vi "viewer.vi"() -> ()   [LabVIEW 2018]
uses:
  Status.ctl
  <vilib>/vision/Avi.llb/IMAQ AVI2 Refnum.ctl
  <vilib>/vision/Image Controls.llb/IMAQ Image.ctl
  Temp/gpm_realsense_videos/Converted/ROI STYP.ctl
  <userlib>/Jet Engineering/JET_QSM/Code/Private/JET_QSM_InvalidOption STYP.ctl
  <vilib>/vision/Avi.llb/IMAQ AVI2 Codec Path.ctl
  <userlib>/Jet Engineering/JET_QSM/Code/Private/JET_QSM - Add State [String API].vi
  <userlib>/Jet Engineering/JET_QSM/Code/Private/JET_QSM - Add State to Front [String API].vi
  <vilib>/Utility/error.llb/Trim Whitespace.vi
  <vilib>/Utility/error.llb/Error Cluster From Error Code.vi
  <vilib>/vision/NI_Vision_Development_Module.lvlib
panel:
  in  "Filter Parameters":T1={"Sigma"=1.0, "HThresh"=0.7, "LThres"=0.2, "WindowSize"=9} {"LThres" min=0 max=1 format="%.2f"; "HThresh" min=0 max=1 format="%.2f"; "Sigma" min=0 max=1 format="%.2f"}
  out "Waveform Graph":u32[][](graph)
  in  "Adjust Filtering Options":bool
  in  "Loop?":bool
  in  "Apply Filtering?":bool
  in  "select roi":bool
  in  "ROI Type":T2
  in  "Exit":bool
  out "playback position":dbl(slide) scale=0.0..100.0
  in  "stop":bool
  in  "Start?":bool
  out "Image":T3(plugin-control)
  in  "Video Path":path
  out "Recent states before Error (with tick counts) 2":string="0.167 sec ago: VI Initialize\n0.167 sec ago: Window Open\n0.110 sec ago: Control Update\n0.110 sec ago: Indicator Update\n0.000 sec ago: Error Handler\r\n"
  in  "Status":T4={"VI"={"error"={"status"=FALSE, "code"=0, "source"=""}, "isExiting?"=FALSE}, "UserLoggedIn?"=FALSE, "AVI Refnum"=refnum, "video path"=path "", "Frame Data"={"Width"=0, "Height"=0, "Frames Per Second"=0, "Codec"="", "Has Data"=FALSE}, "Number of Frames"=0, "Frame Number"=0, "Image Placeholder"=refnum, "Image Output"=refnum, "First Frame?"=TRUE, "Running?"=FALSE, "ROI Type"=enum."Line ROI", "ROI Descriptor"={"Global Rectangle"=[], "Contours"=[]}, "ROI Present?"=FALSE, "Filter Set?"=FALSE, "Loop?"=FALSE, "Filtering?"=FALSE, "Filter Parameters"={"Sigma"=1.0, "HThresh"=0.7, "LThres"=0.2, "WindowSize"=9}} {"Filter Parameters"."LThres" min=0 max=1 format="%.2f"; "Filter Parameters"."HThresh" min=0 max=1 format="%.2f"; "Filter Parameters"."Sigma" min=0 max=1 format="%.2f"; "ROI Descriptor"."Contours"."Type" items=["No Selection", "Point", "Line", "Rectangle", "Oval", "Polygon", "Freehand Region", "Annulus", "Unused2", "Unused3", "Broken Line", "Freehand Line", "Rotated Rectangle"]}
  out "error out":errorcluster
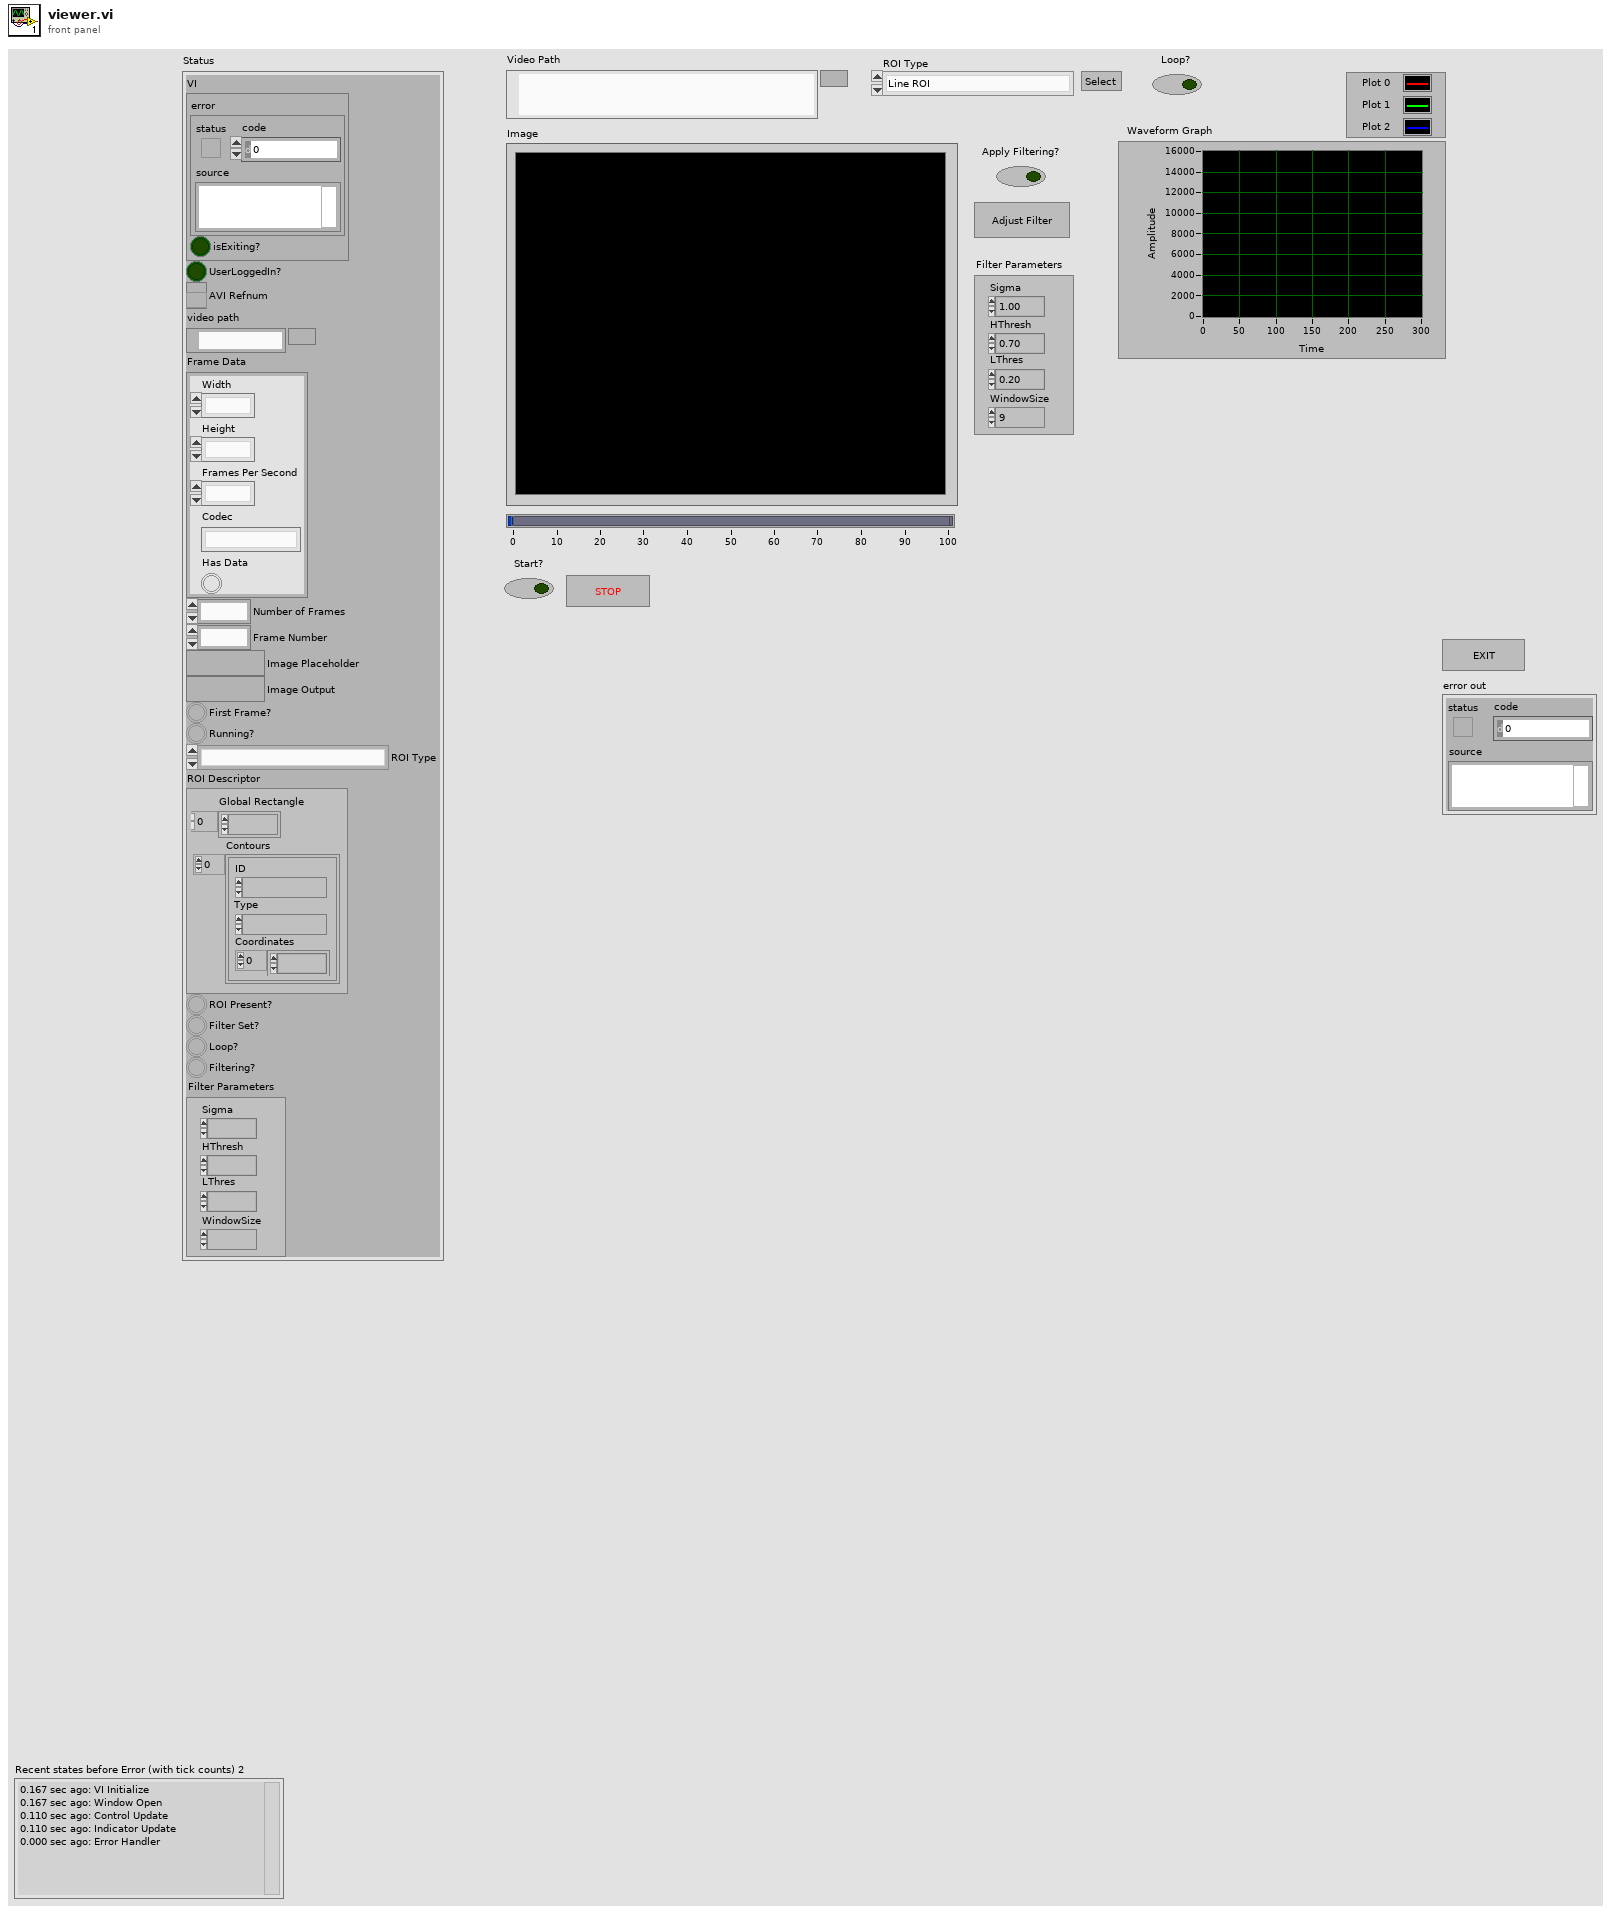
[diagram p1: front panel]
types:
  T1 = cluster{"Sigma":sgl, "HThresh":sgl, "LThres":sgl, "WindowSize":i32}
  T2 = typedef "ROI STYP.ctl" = enum16{"Line ROI", "Rectangle ROI", "Freeform ROI"}
  T3 = typedef "IMAQ Image.ctl" = refnum<image>
  T4 = typedef "Status.ctl" = cluster{"VI":cluster{"error":errorcluster, "isExiting?":bool}, "UserLoggedIn?":bool, "AVI Refnum":T5, "video path":path, "Frame Data":cluster{"Width":u32, "Height":u32, "Frames Per Second":u32, "Codec":string, "Has Data":bool}, "Number of Frames":i32, "Frame Number":u32, "Image Placeholder":T3, "Image Output":T3, "First Frame?":bool, "Running?":bool, "ROI Type":T2, "ROI Descriptor":T6, "ROI Present?":bool, "Filter Set?":bool, "Loop?":bool, "Filtering?":bool, "Filter Parameters":cluster{"Sigma":sgl, "HThresh":sgl, "LThres":sgl, "WindowSize":i32}}
  T5 = typedef "IMAQ AVI2 Refnum.ctl" = refnum<k20>
  T6 = typedef "ROI Descriptor" = cluster{"Global Rectangle":i32[], "Contours":cluster{"ID":enum32{"External", "Internal"}, "Type":u32, "Coordinates":i32[]}[]}
  T7 = typedef "JET_QSM_InvalidOption STYP.ctl" = enum16{"Ignore", "Dialog", "Error"}
  T8 = typedef "JET_QSM_Refnum STYP.ctl" = cluster{"state":cluster{"queue":refnum<queue>, "idle":string, "error":string, "STOP":string}, "debug":cluster{"enabled?":bool, "queue":refnum<queue>}, "Invalid.option":T7, "QSM.Name":string}
  T9 = enum32{"invalid app kind", "Development System", "Run Time System", "Student Edition", "Embedded LabVIEW", "Evaluation", "Custom"}
  T10 = typedef "JET_QSM_Element STYP.ctl" = cluster{"state":string, "data":variant, "comment":string}
  T11 = typedef "IMAQ AVI2 Codec Path.ctl" = u32
  T12 = typedef "Image Type" = u32
  T13 = cluster{"Width":u32, "Height":u32, "Frames Per Second":u32, "Codec":string, "Has Data":bool}
  T14 = typedef "IMAQ Line" = cluster{"Start X":i32, "Start Y":i32, "End X":i32, "End Y":i32}
  T15 = typedef "IMAQ Rectangle" = cluster{"Left":i32, "Top":i32, "Right":i32, "Bottom":i32, "Rotation":dbl}
  T16 = typedef "IMAQ Circle" = cluster{"Center X":i32, "Center Y":i32, "Inner Radius":i32, "Outer Radius":i32, "Start Angle":dbl, "End Angle":dbl}
  T17 = cluster{"Starting Value":sgl, "Incremental Value":sgl, "Histogram":u32[]}
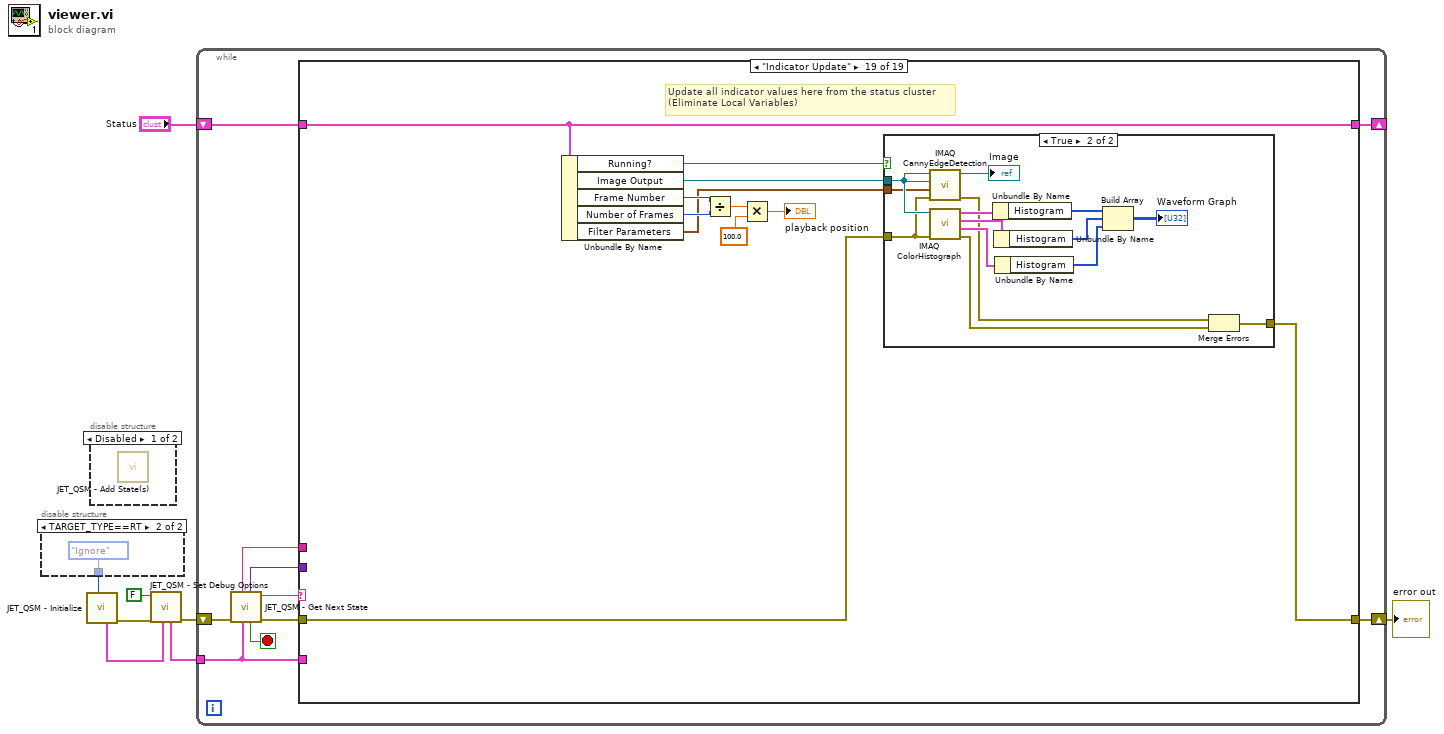
[diagram p0: block diagram]
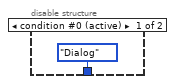
[diagram p2: hidden frame]
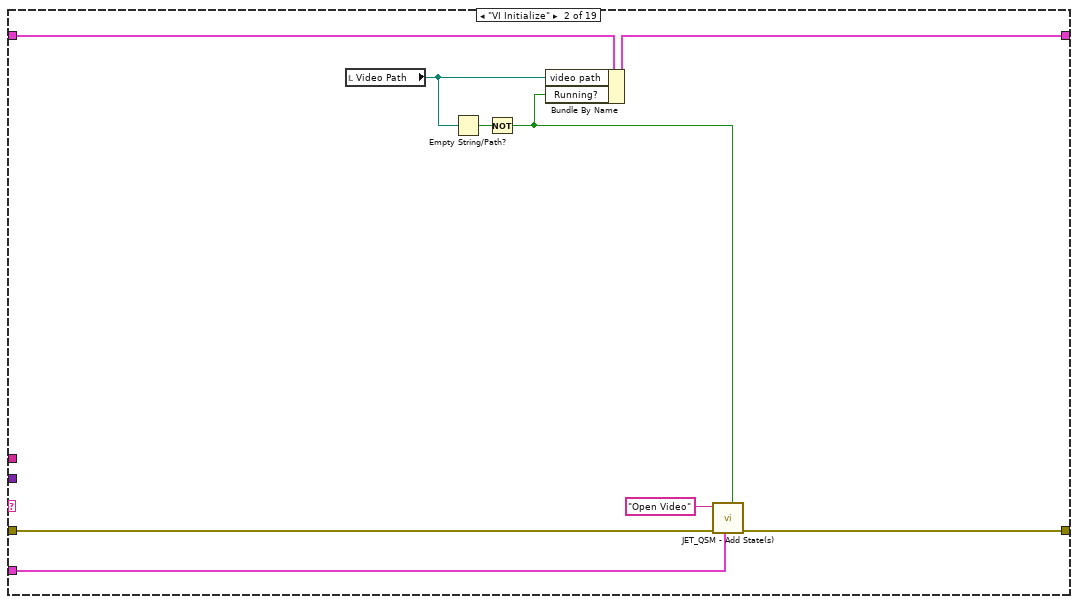
[diagram p5: hidden frame]
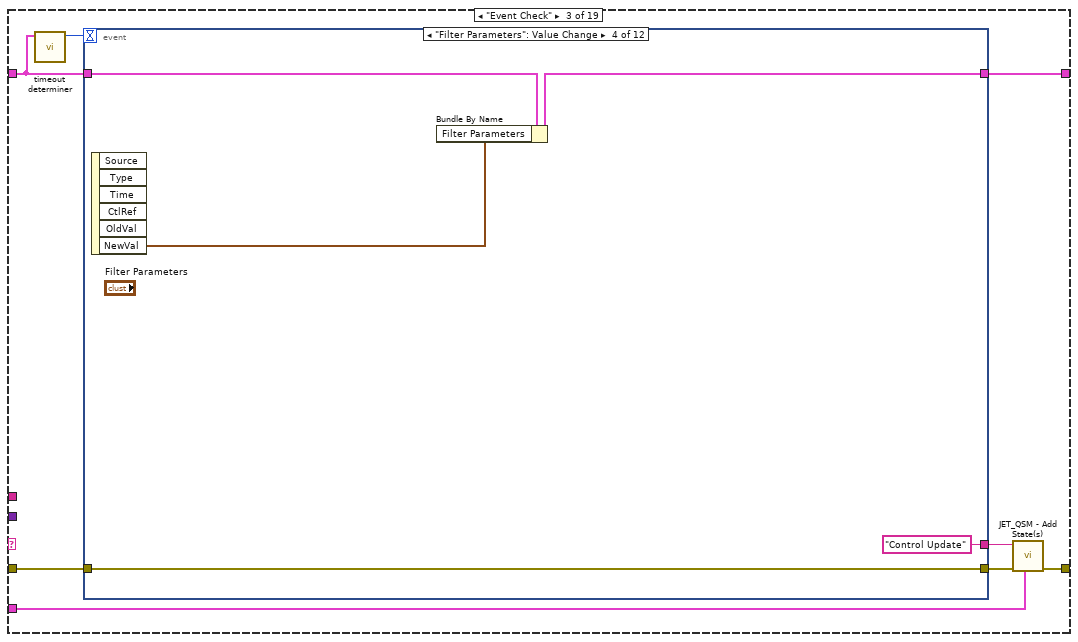
[diagram p6: hidden frame]
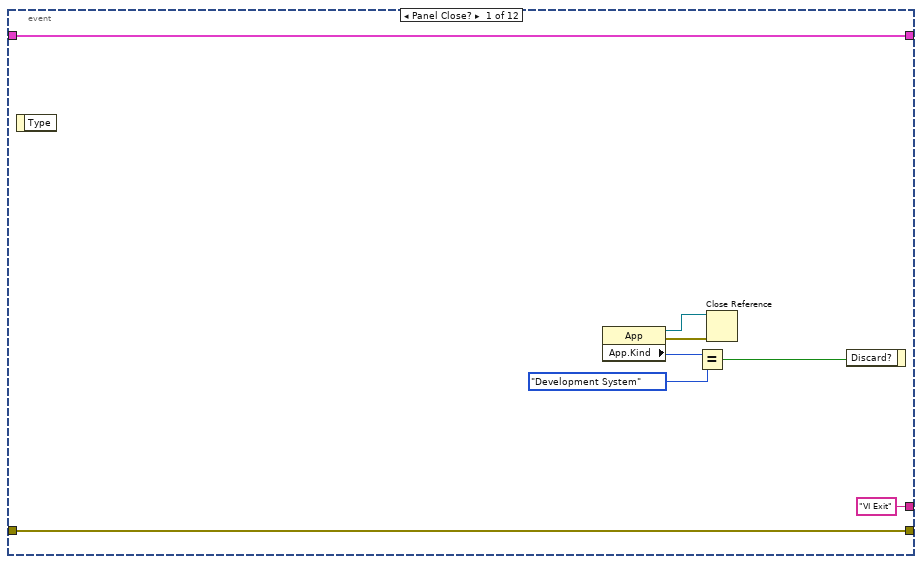
[diagram p7: hidden frame]
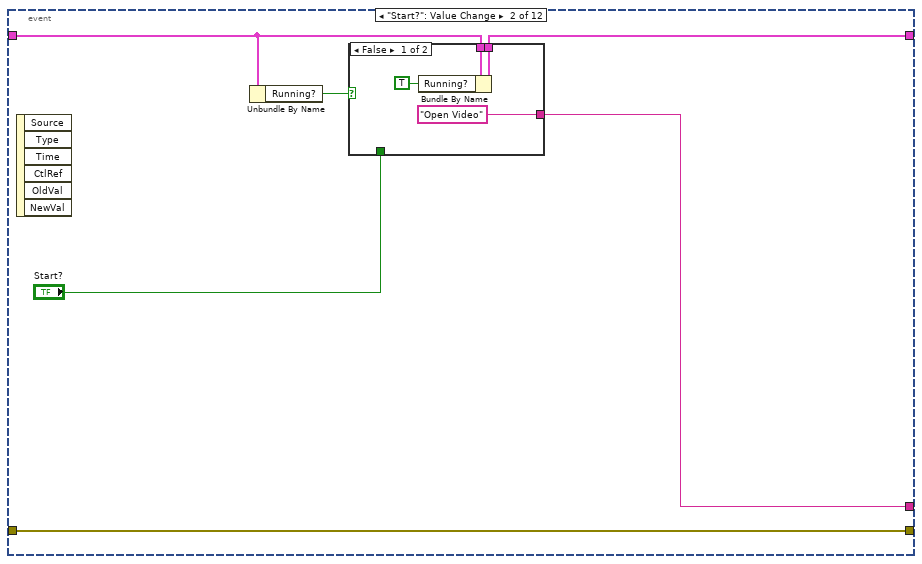
[diagram p8: hidden frame]
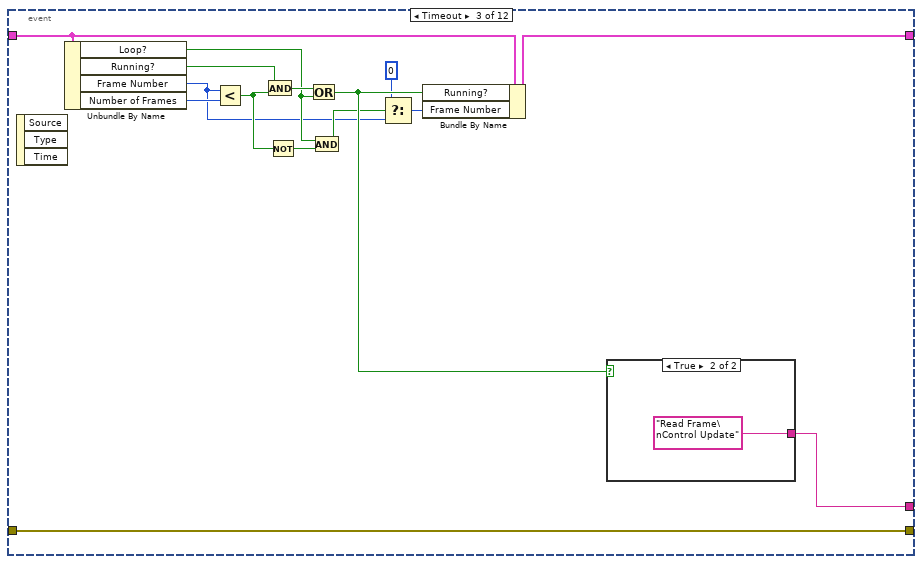
[diagram p10: hidden frame]
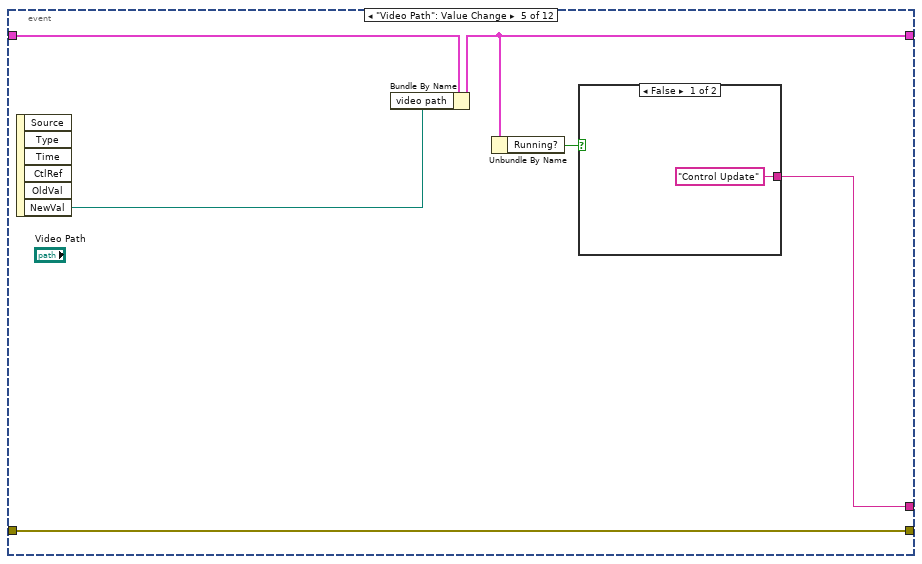
[diagram p12: hidden frame]
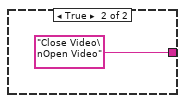
[diagram p13: hidden frame]
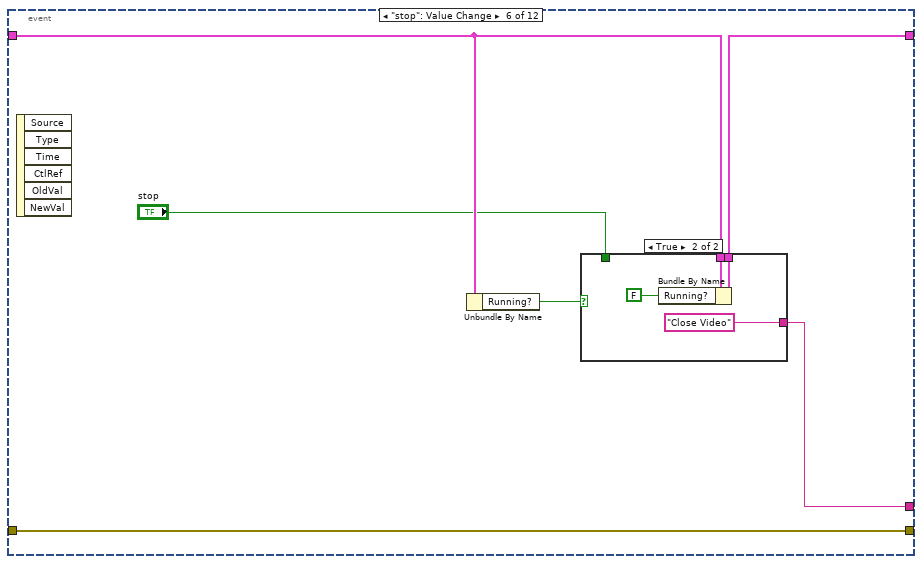
[diagram p14: hidden frame]
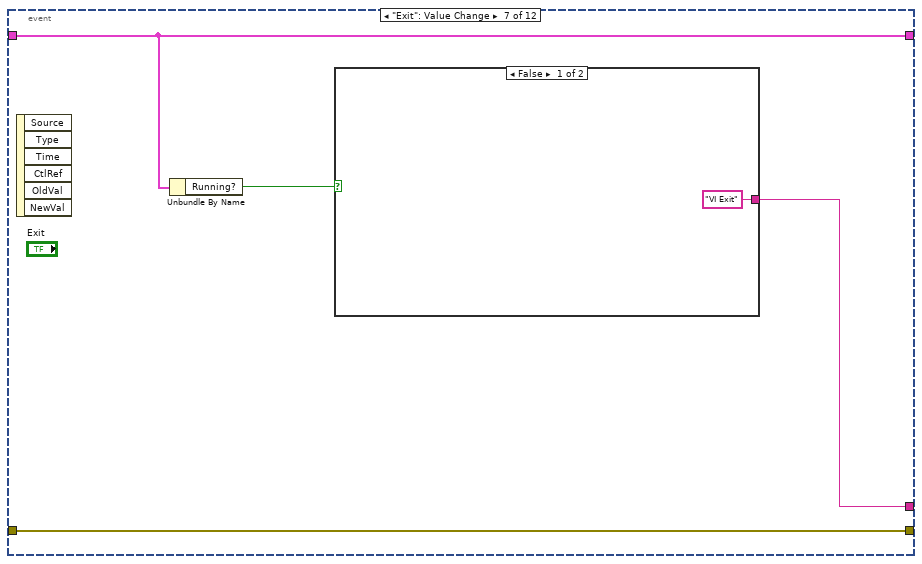
[diagram p16: hidden frame]
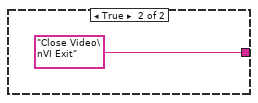
[diagram p17: hidden frame]
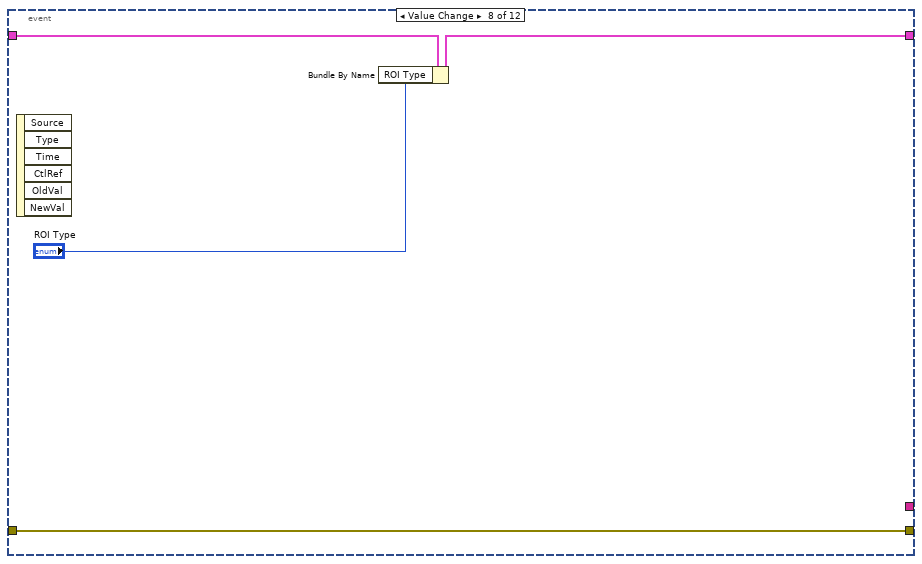
[diagram p18: hidden frame]
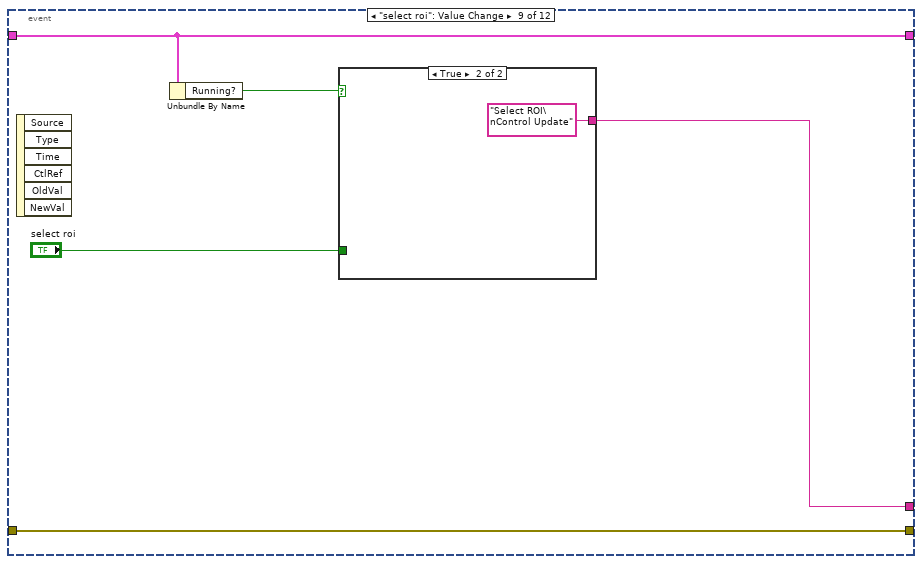
[diagram p19: hidden frame]
diagram:
  n1 = disable-structure shown="TARGET_TYPE==RT" {
    disable-tunnel: [JET_QSM_InvalidOption_STYP."Dialog" ("invalid state action (Dialog)") JET_QSM_InvalidOption_STYP."Ignore" ("invalid state action (Dialog)")] -> w8
    frame condition #0 (active) {
    }
    frame condition #1 {
    }
  }
  n2 = call <userlib>:"JET_QSM - Initialize.vi"("invalid state action (Dialog)"=w8) -> ("error out"=w1:errorcluster, "Jet_QSM refnum"=w4:T8)  [unwired: 9 in]
  n3 = disable-structure shown="Disabled" {
    frame Disabled {
      n4 = call-poly <userlib>:"JET_QSM - Add State(s).vi"() -> ()  [unwired: 11 in, 1 out]
    }
    frame Enabled {
    }
  }
  n5 = call <userlib>:"JET_QSM - Set Debug Options.vi"("Jet_QSM refnum"=w4, "error in (no error)"=w1, "debug.enabled? (F)"=FALSE) -> ("error out"=w2:errorcluster, "Jet_QSM ref"=w3:T8)  [unwired: 7 in]
  n6 = while {
    tunnel: w3 -> [w16]
    shift-right: [w14] -> _
    shift-left: "Status" -> [w15]
    shift-right: [w13] -> w7
    shift-left: w2 -> [w20]
    stop <- w17 stop-if-true
    n7 = call <userlib>:"JET_QSM - Get Next State.vi"("Jet_QSM refnum"=w16, "error in (no error)"=w20) -> ("error out"=w19:errorcluster, "state"=w18:string, "Stop Loop?"=w17:bool, "state data"=w12:variant, "state comment"=w11:string)  [unwired: 5 in]
    n8 = case shown="\"Indicator Update\"" w18 {
      selector: w18 -> [_ _ _ _ _ _ w180 _ _ _ _ _ _ _ _ _ _ _ _]
      tunnel: w19 -> [w21 w31 w39 w141 w172 _ w181 w183 w185 w187 w205 w209 w225 w233 w261 w266 w268 w274 w278]
      tunnel: w16 -> [_ w29 w38 w146 w170 _ w179 _ _ _ _ w210 _ _ _ _ _ w275 _]
      tunnel: w15 -> [w22 w27 w32 w142 w168 w176 w182 w184 w186 w188 w203 w212 w228 w235 w265 w267 w269 w272 w287]
      tunnel: [w22 w26 w34 w140 w168 w176 w182 w184 w186 w188 w202 w211 w228 w231 w264 w267 w269 w272 w287] -> w14
      tunnel: [w21 w30 w36 w147 w172 w177 w178 w183 w185 w187 w195 w207 w224 w234 w259 w266 w268 w273 w279] -> w13
      tunnel: w12 -> [_ _ _ _ _ _ _ _ _ _ _ _ _ _ _ _ _ _ _]
      tunnel: w11 -> [_ _ _ _ _ _ _ _ _ _ _ _ _ _ _ _ _ _ _]
      frame "------ Standard States ------" {
        # "Standard States are required states for a JET_QSM State Machine\n\nTheir names may be changed; use the Initialize function to specify the new names"
        # "This is a section header; the state is never expected to execute"
      }
      frame "VI Initialize" {
        n9 = local read "Video Path"() -> (w25:path)
        n10 = Empty String/Path?(string/path=w25) -> (empty?=w24:bool)
        n11 = Not(x=w24) -> (.not. x?=w23:bool)
        n12 = Bundle By Name(cluster=w27, "video path"=w25, "Running?"=w23) -> (w26:T4)
        n13 = call-poly <userlib>:"JET_QSM - Add State(s).vi"("act? (T)"=w23, "Jet_QSM refnum"=w29, "error in (no error)"=w31, "state(s)"="Open Video") -> ("error out"=w30:errorcluster)  [unwired: 7 in]
      }
      frame "Event Check" {
        n14 = call "timeout determiner.vi"("Status"=w32) -> ("Numeric"=w33:i32)  [unwired: 10 in]
        n15 = event shown="[3] \"Filter Parameters\": Value Change" {
          selector: _ -> [_ _ _ _ _ _ _ _ _ _ _ _]
          dyn-events: _ -> [_ _ _ _ _ _ _ _ _ _ _ _]
          timeout: w33 -> [_ _ _ _ _ _ _ _ _ _ _ _]
          tunnel: w39 -> [w41 w53 w73 w76 w85 w93 w102 w105 w113 w124 w134 w136]
          tunnel: ["VI Exit" ("state(s)") w52 w72 "Control Update" ("state(s)") w80 w91 w99 _ w109 w122 w133 _] -> w37
          tunnel: [w41 w53 w73 w76 w85 w93 w102 w105 w113 w124 w134 w136] -> w35
          tunnel: w32 -> [w40 w50 w69 w79 w84 w90 w101 w108 w112 w117 w129 w139]
          tunnel: [w40 w51 w68 w78 w82 w92 w101 w107 w112 w115 w127 w137] -> w34
          event Panel Close? {
            n16 = event-data() -> ()  [unwired: 1 in, 1 out]
            n17 = property class="App"() -> (reference out=w43:refnum<vi>, error out=w44:errorcluster, "App.Kind"=w47:T9)  [unwired: 2 in]
            n18 = Equal?(x=w47, y=T9."Development System") -> (x = y?=w45:bool)
            n19 = Close Reference(reference=w43, error in (no error)=w44) -> ()  [unwired: 1 out]
            n20 = event-data("Discard?"=w45) -> ()  [unwired: 1 in, 1 out]
          }
          event "Start?": Value Change {
            n21 = event-data() -> ()  [unwired: 1 in, 6 out]
            n22 = Unbundle By Name(w50) -> ("Running?"=w49:bool)
            n23 = case shown="False" w49 {
              tunnel: ["Open Video" ("state(s)") _] -> w52
              tunnel: [w55 w58] -> w51
              tunnel: w50 -> [w54 w58]
              tunnel: "Start?" -> [_ _]
              frame False {
                n24 = Bundle By Name(cluster=w54, "Running?"=TRUE) -> (w55:T4)
              }
              frame True {
              }
            }
          }
          event Timeout {
            n25 = event-data() -> ()  [unwired: 1 in, 3 out]
            n26 = Unbundle By Name(w69) -> ("Loop?"=w65:bool, "Running?"=w70:bool, "Frame Number"=w60:u32, "Number of Frames"=w71:i32)
            n27 = Less?(x=w60, y=w71) -> (x < y?=w64:bool)
            n28 = And(x=w70, y=w64) -> (x .and. y?=w67:bool)
            n29 = Not(x=w64) -> (.not. x?=w63:bool)
            n30 = Or(x=w67, y=w65) -> (x .or. y?=w66:bool)
            n31 = And(x=w65, y=w63) -> (x .and. y?=w61:bool)
            n32 = Select(t=u32 0, s=w61, f=w60) -> (s? t:f=w62:u32)
            n33 = Bundle By Name(cluster=w69, "Running?"=w66, "Frame Number"=w62) -> (w68:T4)
            n34 = case shown="True" w66 {
              tunnel: [_ "Read Frame\nControl Update" ("state(s)")] -> w72
              frame False {
              }
              frame True {
              }
            }
          }
          event "Filter Parameters": Value Change {
            n35 = event-data() -> ("NewVal"=w77:T1)  [unwired: 1 in, 5 out]
            n36 = Bundle By Name(cluster=w79, "Filter Parameters"=w77) -> (w78:T4)
          }
          event "Video Path": Value Change {
            n37 = event-data() -> ("NewVal"=w83:path)  [unwired: 1 in, 5 out]
            n38 = Bundle By Name(cluster=w84, "video path"=w83) -> (w82:T4)
            n39 = Unbundle By Name(w82) -> ("Running?"=w81:bool)
            n40 = case shown="False" w81 {
              tunnel: ["Control Update" "Close Video\nOpen Video"] -> w80
              frame False {
              }
              frame True {
              }
            }
          }
          event "stop": Value Change {
            n41 = event-data() -> ()  [unwired: 1 in, 6 out]
            n42 = Unbundle By Name(w90) -> ("Running?"=w89:bool)
            n43 = case shown="True" w89 {
              tunnel: w90 -> [w94 w98]
              tunnel: [w94 w97] -> w92
              tunnel: [_ "Close Video" ("state(s)")] -> w91
              tunnel: "stop" -> [_ _]
              frame False {
              }
              frame True {
                n44 = Bundle By Name(cluster=w98, "Running?"=FALSE) -> (w97:T4)
              }
            }
          }
          event "Exit": Value Change {
            n45 = event-data() -> ()  [unwired: 1 in, 6 out]
            n46 = Unbundle By Name(w101) -> ("Running?"=w100:bool)
            n47 = case shown="False" w100 {
              tunnel: ["VI Exit" "Close Video\nVI Exit"] -> w99
              frame False {
              }
              frame True {
              }
            }
          }
          event Value Change {
            n48 = event-data() -> ()  [unwired: 1 in, 6 out]
            n49 = Bundle By Name(cluster=w108, "ROI Type"="ROI Type") -> (w107:T4)
          }
          event "select roi": Value Change {
            n50 = event-data() -> ()  [unwired: 1 in, 6 out]
            n51 = Unbundle By Name(w112) -> ("Running?"=w111:bool)
            n52 = case shown="True" w111 {
              tunnel: "select roi" -> [_ _]
              tunnel: [_ "Select ROI\nControl Update"] -> w109
              frame False {
              }
              frame True {
              }
            }
          }
          event "Apply Filtering?": Value Change {
            n53 = event-data() -> ()  [unwired: 1 in, 6 out]
            n54 = Unbundle By Name(w117) -> ("Running?"=w120:bool, "Filter Set?"=w123:bool)
            n55 = And(x=w120, y="Apply Filtering?") -> (x .and. y?=w116:bool)
            n56 = Not(x=w123) -> (.not. x?=w121:bool)
            n57 = Compound Arithmetic op=AND(w120, w121, "Apply Filtering?") -> (w118:bool)
            n58 = Bundle By Name(cluster=w117, "Filtering?"=w116) -> (w115:T4)
            n59 = case shown="True" w118 {
              tunnel: ["Control Update" "Create Filter\nControl Update"] -> w122
              frame False {
              }
              frame True {
              }
            }
          }
          event "Adjust Filtering Options": Value Change {
            n60 = event-data() -> ()  [unwired: 1 in, 6 out]
            n61 = Unbundle By Name(w129) -> ("Running?"=w131:bool, "Filtering?"=w132:bool)
            n62 = And(x=w131, y=w132) -> (x .and. y?=w130:bool)
            n63 = case shown="True" w130 {
              tunnel: [_ "Create Filter\nControl Update" ("state(s)")] -> w133
              frame False {
              }
              frame True {
              }
            }
            n64 = Bundle By Name(cluster=w129, "Filter Set?"=TRUE) -> (w127:T4)
          }
          event "Loop?": Value Change {
            n65 = event-data() -> ("NewVal"=w138:bool)  [unwired: 1 in, 5 out]
            n66 = Bundle By Name(cluster=w139, "Loop?"=w138) -> (w137:T4)
          }
        }
        n67 = call-poly <userlib>:"JET_QSM - Add State(s).vi"("Jet_QSM refnum"=w38, "error in (no error)"=w35, "state(s)"=w37) -> ("error out"=w36:errorcluster)  [unwired: 8 in]
      }
      frame "Error Handler" {
        # "Add specific error exception handlers here"
        n68 = Get Date/Time In Seconds() -> (seconds since 1Jan1904=w150:timestamp)
        n69 = call <userlib>:"JET_QSM - Flush Debug Queue.vi"("Jet_QSM refnum"=w146) -> ("QSM Elements"=w148:T10[], "Timestamps"=w149:timestamp[])  [unwired: 8 in, 1 out]
        n70 = Bundle By Name(cluster=w142, "VI.error"=w141) -> (w140:T4)
        n71 = Unbundle By Name(w141) -> ("code"=w143:i32)
        n72 = for {
          tunnel: w148 -> [w162] mode=indexing
          tunnel: [w160] -> w152 mode=indexing
          tunnel: w150 -> [w157]
          tunnel: w149 -> [w158] mode=indexing
          n73 = Subtract(x=w157, y=w158) -> (x-y=w156:dbl)
          n74 = To Double Precision Float(number=w156) -> (double precision float=w155:dbl)
          n75 = Unbundle By Name(w162) -> ("state"=w161:string)
          n76 = Format Into String(format string="%.03f sec ago: %s", w155, w161) -> (resulting string=w160:string)  [unwired: 2 in, 1 out]
        }
        n77 = case shown="Default" w143 {
          selector: w143 -> [w164]
          tunnel: [w165] -> w144
          tunnel: w141 -> [w163]
          frame Default {
            w165 = TRUE  # Exit?
            n78 = disable-structure shown="Default" {
              disable-tunnel: w164 -> [w167 _]
              disable-tunnel: w163 -> [w166 _]
              frame condition #0 (active) {
                n79 = call <vilib>:"Simple Error Handler.vi"("error code (no error:0)"=w167, "error in (no error)"=w166) -> ()  [unwired: 3 in, 5 out]
              }
              frame condition #1 {
              }
            }
          }
        }
        n80 = Array To Spreadsheet String(delimiter (Tab)="\n", array=w152, 3:"%s" ("format string")) -> (spreadsheet string=→"Recent states before Error (with tick counts) 2":string)
        n81 = call-poly <userlib>:"JET_QSM - Add State(s).vi"("act? (T)"=w144, "Jet_QSM refnum"=w146, "state(s)"="VI Exit") -> ("error out"=w147:errorcluster)  [unwired: 8 in]
      }
      frame "VI Exit" {
        n82 = flat-sequence {
          tunnel: w172 -> [w175]
          tunnel: [w174] -> w171
          tunnel: w170 -> [w173]
          tunnel: [w173] -> w169
          frame #0 {
            n83 = call <userlib>:"JET_QSM - Flush.vi"("Jet_QSM ref"=w173, "error in (no error)"=w175) -> ("error out"=w174:errorcluster)  [unwired: 8 in, 1 out]
          }
        }
        n84 = call <userlib>:"JET_QSM - Add STOP.vi"("Jet_QSM refnum"=w169, "error in (no error)"=w171) -> ()  [unwired: 9 in, 1 out]
      }
      frame "VI STOP" {
        # "Pass out any error that was cached"
        # "This State is the STOP State.\nIt ALWAYS is the last state to execute."
        n85 = Unbundle By Name(w176) -> ("VI.error"=w177:errorcluster)
      }
      frame "INVALID STATE", Default {
        # "This is the state that handles a state name that is INVALID (there is no state for it in the state machine)"
        n86 = call <userlib>:"JET_QSM - INVALID State.vi"("Jet_QSM refnum"=w179, "error in (no error)"=w181, "state"=w180) -> ("error out"=w178:errorcluster)  [unwired: 8 in]
      }
      frame "------ Menu Commands ------" {
        # "This is a section header; the state is never expected to execute"
      }
      frame "------ Events  ------" {
        # "This is a section header; the state is never expected to execute"
      }
      frame "------ Actions  ------" {
        # "This is a section header; the state is never expected to execute"
      }
      frame "Open Video" {
        w190 = T11 1 items=["Default", "System", "Built in Vision"] ("Codec Source")
        n87 = Unbundle By Name(w203) -> ("video path"=w204:path)
        n88 = call "IMAQ AVI2 Open"("error in (no error)"=w205, "Codec Source"=w190, "AVI File Path"=w204) -> ("error out"=w201:errorcluster, "AVI Refnum"=w200:T5)  [unwired: 7 out]
        n89 = call "IMAQ AVI2 Get Info"("error in (no error)"=w201, "AVI Refnum"=w200) -> ("error out"=w196:errorcluster, "Image Type"=w193:T12, "Number of Frames"=w198:u32, "AVI Refnum (duplicate)"=w199:T5, "Frame Data"=w189:T13)  [unwired: 5 out]
        n90 = call "IMAQ Create"("Image Name"="AVI Source", "Image Type"=w193, "error in (no error)"=w196) -> ("New Image"=w192:T3, "error out"=w195:errorcluster)  [unwired: 1 in, 1 out]
        n91 = Bundle By Name(cluster=w203, "Frame Data"=w189, "AVI Refnum"=w199, "Number of Frames"=w198, "First Frame?"=TRUE, "Image Placeholder"=w192, "Frame Number"=u32 0) -> (w202:T4)
      }
      frame "Read Frame" {
        n92 = in-place {
          in-place-border: w209 -> [w220]
          in-place-border: [w219] -> _
          in-place-border: [w213] -> w208
          n93 = in-place-cluster #1(w212) -> ("AVI Refnum"=w221:T5, "Image Placeholder"=w214:T3, "Frame Number"=w217:u32, "ROI Present?"=w213:bool)  [unwired: 1 out]
          n94 = Increment(x=w217) -> (x+1=w216:u32)
          n95 = call "IMAQ AVI2 Read Frame"("error in (no error)"=w220, "Frame Number"=w217, "Image"=w214, "AVI Refnum"=w221) -> ("error out"=w219:errorcluster, "Image Out"=w215:T3, "AVI Refnum (duplicate)"=w218:T5)  [unwired: 5 out]
          n96 = in-place-cluster #1("AVI Refnum"=w218, "Image Placeholder"=w214, "Frame Number"=w216, "Image Output"=w215, "ROI Present?"=w213) -> (w211:T4)
        }
        n97 = call-poly <userlib>:"JET_QSM - Add State(s).vi"("act? (T)"=w208, "Jet_QSM refnum"=w210, "error in (no error)"=w209, "state(s)"="Apply ROI Mask") -> ("error out"=w207:errorcluster)  [unwired: 7 in]
      }
      frame "Close Video" {
        n98 = Unbundle By Name(w228) -> ("AVI Refnum"=w226:T5, "Image Placeholder"=w227:T3)
        n99 = call "IMAQ AVI2 Close"("AVI Refnum"=w226) -> ("error out"=w222:errorcluster)  [unwired: 1 in, 9 out]
        n100 = call "IMAQ Dispose"("Image"=w227) -> ("error out"=w223:errorcluster)  [unwired: 2 in, 3 out]
        n101 = Merge Errors(w223, w222, w225) -> (w224:errorcluster)
      }
      frame "Select ROI" {
        n102 = Unbundle By Name(w235) -> ("ROI Type"=w237:T2, "Image Output"=w236:T3)
        n103 = case shown="\"Line ROI\", Default" w237 {
          tunnel: w236 -> [w244 w251 w257]
          tunnel: w233 -> [w243 w250 w256]
          tunnel: [w240 w246 w255] -> w234
          tunnel: [w239 w249 w253] -> w232
          tunnel: [w238 w245 w252] -> w230
          frame "Line ROI", Default {
            n104 = call "IMAQ Select Line"("error in (no error)"=w243, "Image In"=w244) -> ("error out"=w241:errorcluster, "Cancelled"=w238:bool, "Line"=w242:T14)  [unwired: 6 in, 1 out]
            n105 = call "IMAQ Convert Line to ROI"("error in (no error)"=w241, "Line"=w242) -> ("error out"=w240:errorcluster, "ROI Descriptor"=w239:T6)  [unwired: 7 in]
          }
          frame "Rectangle ROI" {
            n106 = call "IMAQ Select Rectangle"("error in (no error)"=w250, "Image In"=w251) -> ("error out"=w247:errorcluster, "Cancelled"=w245:bool, "Rectangle"=w248:T15)  [unwired: 6 in, 1 out]
            n107 = call "IMAQ Convert Rectangle to ROI"("error in (no error)"=w247, "Rectangle"=w248) -> ("error out"=w246:errorcluster, "ROI Descriptor"=w249:T6)  [unwired: 7 in]
          }
          frame "Freeform ROI" {
            n108 = call "IMAQ Select Annulus"("error in (no error)"=w256, "Image In"=w257) -> ("error out"=w255:errorcluster, "Cancelled"=w252:bool, "Annulus"=w254:T16)  [unwired: 6 in, 1 out]
            n109 = call "IMAQ Convert Annulus to ROI"("error in (no error)"=w255, "Annulus"=w254) -> ("ROI Descriptor"=w253:T6)  [unwired: 7 in, 1 out]
          }
        }
        n110 = Not(x=w230) -> (.not. x?=w229:bool)
        n111 = Bundle By Name(cluster=w235, "ROI Descriptor"=w232, "ROI Present?"=w229) -> (w231:T4)
      }
      frame "Apply ROI Mask" {
        n112 = Unbundle By Name(w265) -> ("Image Output"=w263:T3, "ROI Descriptor"=w262:T6)  [unwired: 1 out]
        n113 = call "IMAQ Overlay ROI"("error in (no error)"=w261, "Point Symbol"=u32[][] [[16711681, 16777216, 16777216, 0, 16777216, 16777216, 16777216], [16777216, 16777216, 16777216, 0, 16777216, 16777216, 16777216], [16777216, 16777216, 16777216, 0, 16777216, 16777216, 16777216], [0, 0, 0, 16777216, 0, 0, 0], [16777216, 16777216, 16777216, 0, 16777216, 16777216, 16777216], [16777216, 16777216, 16777216, 0, 16777216, 16777216, 16777216], [16777216, 16777216, 16777216, 0, 16777216, 16777216, 16777216]], "ROI Descriptor"=w262, "Image"=w263) -> ("error out"=w259:errorcluster, "Image Out"=w260:T3)  [unwired: 6 in]
        n114 = Bundle By Name(cluster=w265, "Image Output"=w260) -> (w264:T4)
      }
      frame "Create Filter" {
      }
      frame "------ Window and Panel Control ------" {
        # "This is a section header; the state is never expected to execute"
      }
      frame "Control Update" {
        # "Update all control properties here from the status cluster\n(Consolidate/reduce property nodes)"
        n115 = Unbundle By Name(w272) -> ("Loop?"=w271:bool, "Filter Parameters"=w270:T1)  [unwired: 1 out]
        n116 = local write "Filter Parameters"(w270) -> ()
        n117 = local write "Loop?"(w271) -> ()
        n118 = call-poly <userlib>:"JET_QSM - Add State(s).vi"("Jet_QSM refnum"=w275, "error in (no error)"=w274, "state(s)"="Indicator Update") -> ("error out"=w273:errorcluster)  [unwired: 8 in]
      }
      frame "Indicator Update" {
        # "Update all indicator values here from the status cluster\n(Eliminate Local Variables)"
        n119 = Unbundle By Name(w287) -> ("Running?"=w280:bool, "Image Output"=w281:T3, "Frame Number"=w285:u32, "Number of Frames"=w286:i32, "Filter Parameters"=w277:T1)
        n120 = Divide(x=w285, y=w286) -> (x/y=w284:dbl)
        n121 = Multiply(x=w284, y=100.0) -> (x*y=→"playback position":dbl)
        n122 = case shown="True" w280 {
          tunnel: w281 -> [_ w295]
          tunnel: [w288 w292] -> w279
          tunnel: w278 -> [w288 w293]
          tunnel: w277 -> [_ w289]
          frame False {
          }
          frame True {
            n123 = call "IMAQ CannyEdgeDetection"("Image Src"=w295, "Image Dst"=w295, "Filter Parameters"=w289, "error in (no error)"=w293) -> ("Image Dst Out"=→"Image":T3, "error out"=w291:errorcluster)  [unwired: 4 in]
            n124 = call "IMAQ ColorHistograph"("Image Src"=w295, "error in (no error)"=w293) -> ("Red or Hue Histogram Graph"=w302:T17, "Green or Sat Histogram Graph"=w301:T17, "Blue or Luma or Val or Inten Histogram Graph"=w300:T17, "error out"=w290:errorcluster)  [unwired: 4 in]
            n125 = Unbundle By Name(w302) -> ("Histogram"=w299:u32[])
            n126 = Unbundle By Name(w301) -> ("Histogram"=w298:u32[])
            n127 = Unbundle By Name(w300) -> ("Histogram"=w297:u32[])
            n128 = Build Array(w299, w298, w297) -> (→"Waveform Graph":u32[][])
            n129 = Merge Errors(w291, w290) -> (w292:errorcluster)
          }
        }
      }
    }
  }
  "error out" <- w7
